vi "WSVCAP SHL FPGA LL I2C Procedure - Send Data Byte.vi"(0 "Procedure Step":T1, 1 "Wait Ticks Remaining":u32, 5 "I2C Wait Ticks":u32, 7 "Write Bits Remaining":u8, 11 "error in (no error)":errorcluster, 13 "Socket Mask":u64 format="%012x") -> (3 "Wait Ticks Remaining Out":u32, 4 "Procedure Step Out":T1, 8 "Write Bits Remaining Out":u8, 10 "Finished":bool, 15 "error out":errorcluster)   [LabVIEW 2012]
uses:
  Type Defs/WSVCAP SHL Procedure Step Enum.ctl
  Type Defs/WSVCAP SHL I2C Write Line Enum.ctl
  Type Defs/WSVCAP SHL FIFO Operation Enum.ctl
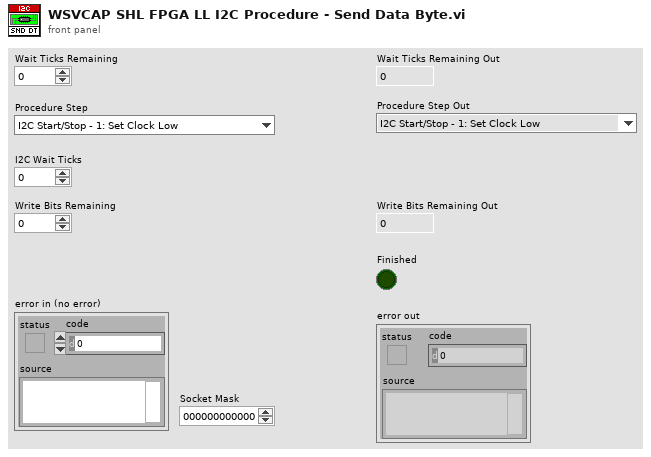
[diagram p1: front panel]
types:
  T1 = typedef "WSVCAP SHL Procedure Step Enum.ctl" = enum16{"I2C Start/Stop - 1: Set Clock Low", "I2C Start/Stop - 2: Wait", "I2C Start/Stop - 3: Set Data I", "I2C Start/Stop - 4: Wait", "I2C Start/Stop - 5: Set Clock High", "I2C Start/Stop - 6: Wait", "I2C Start/Stop - 7: Set Data II", "I2C Start/Stop - 8: Wait", "I2C Start/Stop - 9: Set Clock Low", "I2C Start/Stop - 10: Wait", "I2C Read ACK - 1: Set Clock High", "I2C Read ACK - 2: Wait", "I2C Read ACK - 3: Read ACK Bit", "I2C Read ACK - 4: Wait", "I2C Read ACK - 5: Set Clock Low", "I2C Read ACK - 6: Wait", "I2C Write ACK - 1: Write ACK Bit", "I2C Write ACK - 2: Wait", "I2C Write ACK - 3: Set Clock High", "I2C Write ACK - 4: Wait", "I2C Write ACK - 5: Set Clock Low", "I2C Write ACK - 6: Wait", "I2C Write ACK - 7: Set Data Low", "I2C Send Add - 1: Reset Bits Remaining", "I2C Send Add - 2: Set Data Bit", "I2C Send Add - 3: Wait", "I2C Send Add - 4: Set Clock High", "I2C Send Add - 5: Wait", "I2C Send Add - 6: Set Clock Low", "I2C Send Add - 7: Wait", "I2C Send Add - 8: Check Bits Remaining", "I2C Send Data - 1: Reset Bits Remaining", "I2C Send Data - 2: Load Write Bit from FIFO", "I2C Send Data - 3: Set Data Bit", "I2C Send Data - 4: Wait", "I2C Send Data - 5: Set Clock High", "I2C Send Data - 6: Wait", "I2C Send Data - 7: Set Clock Low", "I2C Send Data - 8: Wait", "I2C Send Data - 9: Check Bits Remaining", "I2C Receive Data - 1: Reset Bits Remaining", "I2C Receive Data - 2: Wait", "I2C Receive Data - 3: Set Clock High", "I2C Receive Data - 4: Wait", "I2C Receive Data - 5: Read Data Bit", "I2C Receive Data - 6: Wait", "I2C Receive Data - 7: Set Clock Low", "I2C Receive Data - 8: Wait", "I2C Receive Data - 9: Check Bits Remaining", "SPI Clear Lines - 1:Clear", "SPI Send/Receive - 1: Load SDA - Clock Low", "SPI Send/Receive - 2: Wait", "SPI Send/Receive - 3: Load DATO - Clock High", "SPI Send/Receive - 4: Wait", "SPI Wait CMD Delay - 1:Wait", "RFFE Send SSC - 1:Set Low", "RFFE Send SSC - 2:Wait", "RFFE Send SSC - 3:Set SDA High", "RFFE Send SSC - 4:Wait", "RFFE Send SSC - 5:Set SDA Low", "RFFE Send SSC - 6:Wait", "RFFE Send Data - 1:Set SCL High", "RFFE Send Data - 2:Wait", "RFFE Send Data - 3:Set SCL Low", "RFFE Send Data - 4:Wait", "RFFE Send Data - 5:Set SCL High (P)", "RFFE Send Data - 6:Wait", "RFFE Send Data - 7:Set SCL Low (P)", "RFFE Send Data - 8:Wait", "RFFE Send Data - 9:Set SCL High (BP)", "RFFE Send Data - 10:Wait", "RFFE Send Data - 11:Set SCL Low (BP)", "RFFE Send Data - 12:Wait", "RFFE Receive Data - 1:Set SCL High", "RFFE Receive Data - 2:Wait", "RFFE Receive Data - 3:Set SCL Low", "RFFE Receive Data - 4:Wait", "RFFE Receive Data - 5:Set SCL High (BP)", "RFFE Receive Data - 6:Wait", "RFFE Receive Data - 7:Set SCL Low (BP)", "RFFE Receive Data - 8:Wait", "RFFE Wait CMD Delay - 1:Wait", "RFFE Clear Lines - 1:Clear"}
  T2 = typedef "WSVCAP SHL I2C Write Line Enum.ctl" = enum16{"I2C SCL", "I2C SDA"}
  T3 = typedef "WSVCAP SHL FIFO Operation Enum.ctl" = enum16{"Create FIFO/Memory", "Get Write FIFO Status", "Get Read FIFO Status", "Put Element in Write", "Put Element in Read", "Get Element from Write", "Get Element from Read"}
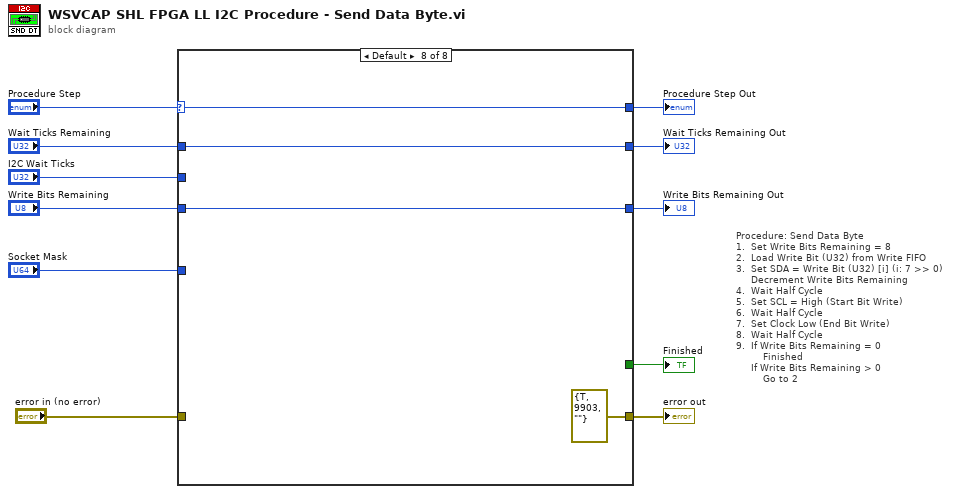
[diagram p0: block diagram]
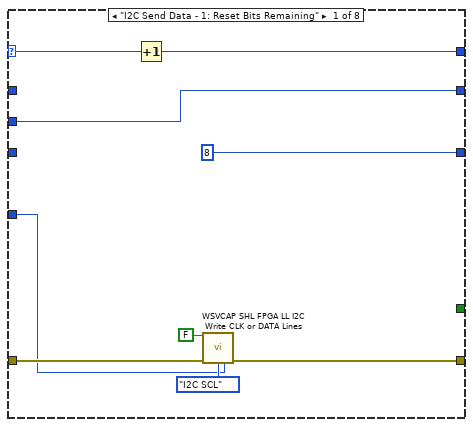
[diagram p2: hidden frame]
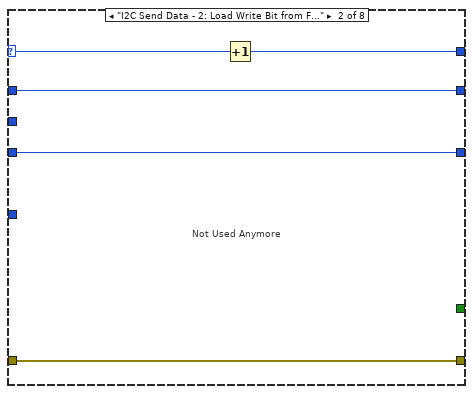
[diagram p3: hidden frame]
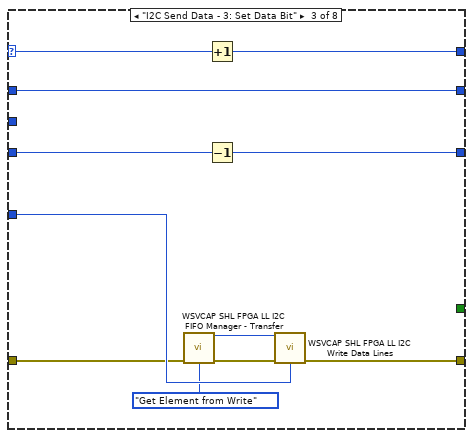
[diagram p4: hidden frame]
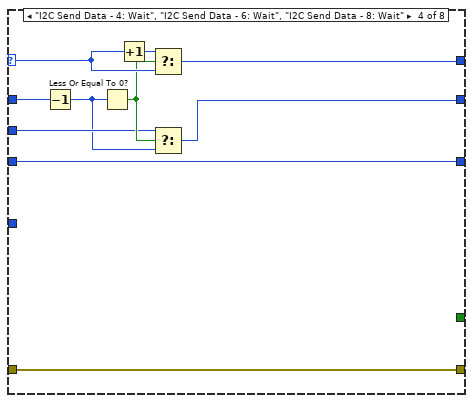
[diagram p5: hidden frame]
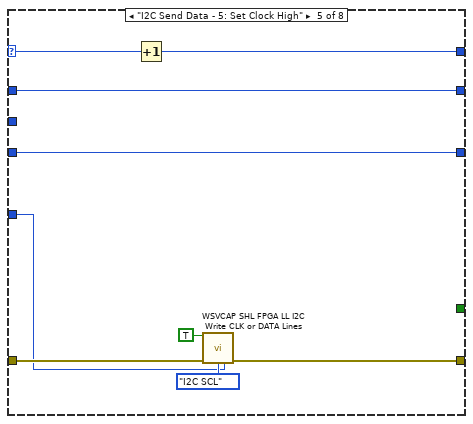
[diagram p6: hidden frame]
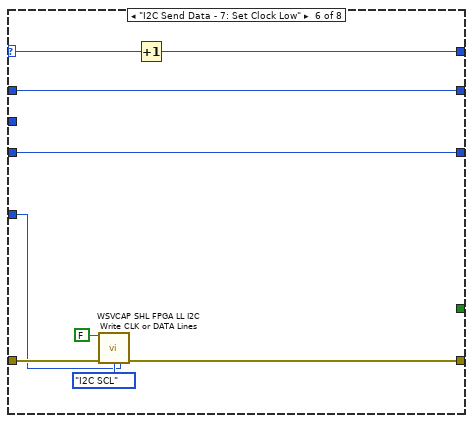
[diagram p7: hidden frame]
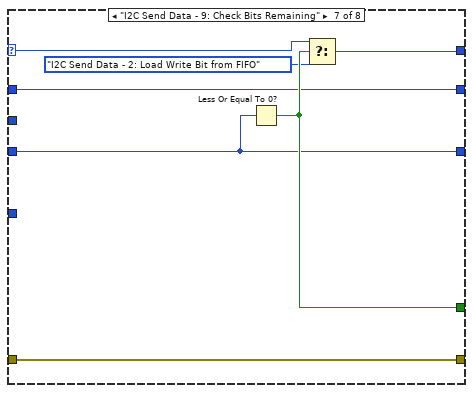
[diagram p8: hidden frame]
diagram:
  # "Procedure: Send Data Byte\n1.  Set Write Bits Remaining = 8\n2.  Load Write Bit (U32) from Write FIFO\n3.  Set SDA = Write Bit (U32) [i] (i: 7 >> 0)\n     Decrement Write Bits Remaining\n4.  Wait Half Cycle\n5.  Set SCL = High (Start Bit Write)\n6.  Wait Half Cycle\n7.  Set Clock Low (End Bit Write)\n8.  Wait Half Cycle\n9.  If Write Bits Remaining = 0\n         Finished\n     If Write Bits Remaining > 0\n         Go to 2"
  n1 = case shown="Default" "Procedure Step" {
    selector: "Procedure Step" -> [w16 w25 w35 w45 w52 w60 w66 w74]
    tunnel: [w18 w21 w36 w43 w53 w62 w71 errorcluster {"status"=TRUE, "code"=9903, "source"=""} ("error IO")] -> w10
    tunnel: "error in (no error)" -> [w19 w21 w31 w43 w54 w63 w71 _]
    tunnel: "Wait Ticks Remaining" -> [_ w23 w26 w46 w48 w57 w65 w73]
    tunnel: "I2C Wait Ticks" -> [w14 _ _ w41 _ _ _ _]
    tunnel: "Write Bits Remaining" -> [_ w22 w34 w37 w47 w56 w67 w72]
    tunnel: [_ _ _ _ _ _ w70 _] -> w9
    tunnel: "Socket Mask" -> [w15 _ w33 _ w50 w59 _ _]
    tunnel: [w14 w23 w26 w39 w48 w57 w65 w73] -> w3
    tunnel: [u8 8 ("Write Bits Remaining") w22 w27 w37 w47 w56 w67 w72] -> w2
    tunnel: [w12 w24 w28 w38 w49 w58 w68 w74] -> w1
    frame "I2C Send Data - 1: Reset Bits Remaining" {
      n2 = Increment(x=w16) -> (x+1=w12:T1)
      n3 = call "WSVCAP SHL FPGA LL I2C Write CLK or DATA Lines.vi"("Bit In"=FALSE, "error in (no error)"=w19, "Line"=WSVCAP_SHL_I2C_Write_Line_Enum."I2C SCL", "Socket Mask"=w15) -> ("error out"=w18:errorcluster)  [unwired: 11 in]
    }
    frame "I2C Send Data - 2: Load Write Bit from FIFO" {
      # "Not Used Anymore"
      n4 = Increment(x=w25) -> (x+1=w24:T1)
    }
    frame "I2C Send Data - 3: Set Data Bit" {
      n5 = call "WSVCAP SHL FPGA LL I2C FIFO Manager - Transfer.vi"("error in (no error)"=w31, "Operation"=WSVCAP_SHL_FIFO_Operation_Enum."Get Element from Write") -> ("Data Out"=w29:u64, "error out"=w30:errorcluster)  [unwired: 11 in, 1 out]
      n6 = Increment(x=w35) -> (x+1=w28:T1)
      n7 = Decrement(x=w34) -> (x-1=w27:u8)
      n8 = call "WSVCAP SHL FPGA LL I2C Write Data Lines.vi"("Write Bit (U64)"=w29, "error in (no error)"=w30, "Socket Mask"=w33) -> ("error out"=w36:errorcluster)  [unwired: 12 in]
    }
    frame "I2C Send Data - 4: Wait", "I2C Send Data - 6: Wait", "I2C Send Data - 8: Wait" {
      n9 = Decrement(x=w46) -> (x-1=w40:u32)
      n10 = Less Or Equal To 0?(x=w40) -> (x <= 0?=w42:bool)
      n11 = Increment(x=w45) -> (x+1=w44:T1)
      n12 = Select(t=w44, s=w42, f=w45) -> (s? t:f=w38:T1)
      n13 = Select(t=w41, s=w42, f=w40) -> (s? t:f=w39:u32)
    }
    frame "I2C Send Data - 5: Set Clock High" {
      n14 = Increment(x=w52) -> (x+1=w49:T1)
      n15 = call "WSVCAP SHL FPGA LL I2C Write CLK or DATA Lines.vi"("Bit In"=TRUE, "error in (no error)"=w54, "Line"=WSVCAP_SHL_I2C_Write_Line_Enum."I2C SCL", "Socket Mask"=w50) -> ("error out"=w53:errorcluster)  [unwired: 11 in]
    }
    frame "I2C Send Data - 7: Set Clock Low" {
      n16 = call "WSVCAP SHL FPGA LL I2C Write CLK or DATA Lines.vi"("Bit In"=FALSE, "error in (no error)"=w63, "Line"=WSVCAP_SHL_I2C_Write_Line_Enum."I2C SCL", "Socket Mask"=w59) -> ("error out"=w62:errorcluster)  [unwired: 11 in]
      n17 = Increment(x=w60) -> (x+1=w58:T1)
    }
    frame "I2C Send Data - 9: Check Bits Remaining" {
      n18 = Less Or Equal To 0?(x=w67) -> (x <= 0?=w70:bool)
      n19 = Select(t=w66, s=w70, f=WSVCAP_SHL_Procedure_Step_Enum."I2C Send Data - 2: Load Write Bit from FIFO" ("Procedure Step")) -> (s? t:f=w68:T1)
    }
    frame Default {
    }
  }
  "error out" <- w10
  "Finished" <- w9
  "Procedure Step Out" <- w1
  "Wait Ticks Remaining Out" <- w3
  "Write Bits Remaining Out" <- w2
